vi "Lvi Select Channels.vi"(6 "MaxRange":dbl, 7 "MinRange":dbl, 8 "error in (no error)":errorcluster, 9 "Gain":u32, 10 "ChanListStr":string, 11 "TaskRef":i32) -> (0 "error out":errorcluster, 1 "function return":u32(ring), 2 "ActualNumChannels":u32, 3 "TaskRef out":i32)   [LabVIEW 2022 SP3, in "DtLvLink.lvlib"]
doc: "Calls directly into the entry points of the DLL of the Data Acq SDK to select channels for use in the task. This VI is used by the higher-level VI, DtOLCreateTask."
uses:
  DtLvLink.lvlib
  <userlib>/LV-Link3/DtLvLink_64.dll
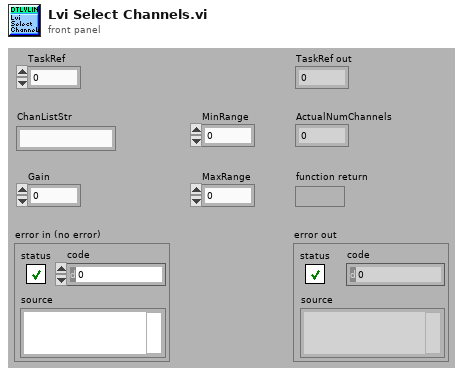
[diagram p1: front panel]
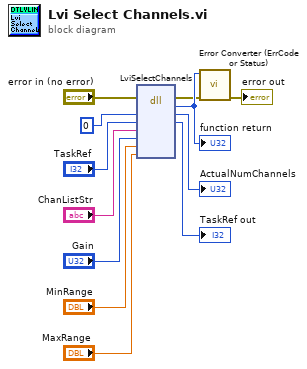
[diagram p0: block diagram]
diagram:
  n1 = dll-call lib="C:/Program Files/National Instruments/LabVIEW 2022/user.lib/LV-Link3/DtLvLink_64.*" fn="LviSelectChannels"(error in="error in (no error)", "ActualNumChannels"=u32 0, "TaskRef"="TaskRef", "ChanListStr"="ChanListStr", "Gain"="Gain", "MinRange"="MinRange", "MaxRange"="MaxRange") -> (error out=w2:errorcluster, w12:u32, "ActualNumChannels"=→"ActualNumChannels":u32, "TaskRef"=→"TaskRef out":i32)  [unwired: 6 in, 1 out]
  "function return" <- w12
  n2 = call "Error Converter (ErrCode or Status).vi"("error in (no error)"=w2, "error code"=w12) -> ("error out"=→"error out":errorcluster)  [unwired: 9 in]
